vi "Enable Remote Sensing.vi"(8 "error in (no error)":errorcluster, 9 "Function (0:Voltage)":u16(ring) items=["Voltage", "Current", "Resistance", "Digitize Voltage", "Digitize Current"], 10 "Enable Remote Sensing (T: Enable)":bool=TRUE, 11 "VISA resource name":refnum<visa-resource-name>) -> (0 "error out":errorcluster, 3 "VISA resource name out":refnum<visa-resource-name>)   [LabVIEW 2015, in "Keithley 2450.lvlib"]
doc: "Enables Remote (4-wire) sensing. This type of sensing allows the instrument to bypass the input and output leads and make a more accurate measurement at the device under test. This also allows the source to adjust its voltage so that the desired voltage is located at the sensing leads, not at the input and output jacks."
uses:
  <instrlib>/Keithley 2450/Keithley 2450.lvlib
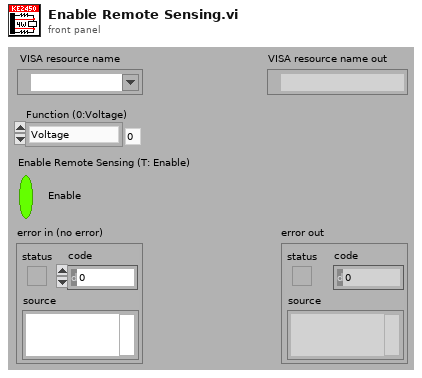
[diagram p1: front panel]
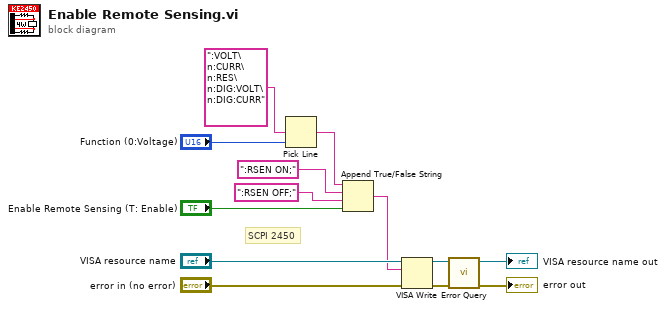
[diagram p0: block diagram]
diagram:
  # "SCPI 2450"
  n1 = Pick Line(multi-line string=":VOLT\n:CURR\n:RES\n:DIG:VOLT\n:DIG:CURR", line index="Function (0:Voltage)") -> (output string=w1:string)  [unwired: 1 in]
  n2 = Append True/False String(1:"Enable Remote Sensing (T: Enable)", 2:":RSEN OFF;", 3:":RSEN ON;", 4:w1) -> (0:w7:string)
  n3 = VISA Write(VISA resource name="VISA resource name", write buffer=w7, error in (no error)="error in (no error)") -> (VISA resource name out=w9:refnum<visa-resource-name>, error out=w8:errorcluster)  [unwired: 1 out]
  n4 = call <instrlib>:"Error Query.vi"("error in (no error)"=w8, "VISA resource name"=w9) -> ("error out"=→"error out":errorcluster, "VISA resource name out"=→"VISA resource name out":refnum<visa-resource-name>)  [unwired: 8 out]
